vi "point-picker.vi"() -> ()   [LabVIEW 2013]
uses:
  <vilib>/Utility/file.llb/Read From Spreadsheet File (DBL).vi
panel:
  out "X Scale.Range:Minor Increment":dbl=0.00010000000000000009
  out "Slice":dbl[](graph)=[0.03882083763653586, 0.036301990430997515, 0.06641265033129048, 0.022599259175726628, 0.03963233726656525, 0.057976093950650155, 0.02605338207009137, 0.04157947175893252, 0.008818364898812232, 0.03339557369538179, 0.009831003676912626, 0.0298513507596618, 0.000720265042160115, 0.04957020405641017, 0.028435297883295477, 0.02968065104257011, 0.054593725454568406, 0.02941844990660442, 0.0016610067970859927, 0.037814320441856994, 0.03162073969486945, 0.04354178631802414, 0.01837108453843325, 0.020494923878462044, 0.02146464095599344, 0.050724892633311223, 0.055113319254019744, 0.010244418203584982, 0.02498233101668227, 0.02800231949963939, 0.02428971264494624, 0.03964718893141746, 0.03696606646661389, 0.04173575239047644, 0.08038701264805279, 0.05693297539500711, 0.031549742745971894, 0.010177653448556319, 0.047274462597502925, 0.018015425707227962, 0.032278808272603966, 0.04953827011027471, 0.06425909702809958, 0.018330341600943854, 0.03463798404659602, 0.03930752357841345, 0.06796427722786236, 0.02058242219084138, 0.04370799015223786, 0.023590787930164128, 0.008461873502233855, 0.029360130887503208, 0.029158674398922235, 0.03945732345450104, 0.012916360547716334, 0.02759490800230026, 0.03753745241666211, 0.028389751605858184, 0.0150134372573898, 0.009742076686166182, 0.019301765168510596, 0.017192190302683024, 0.037235678285443434, 0.011830534813551296, 0.002788759120713905, 0.047997520126393176, 0.030486497700197693, 0.0546373685612716, 0.033694598255554375, 0.07210813163063974, 0.0698476088075215, 0.05675370368842305, 0.018003794508399205, 0.05840152492070653, 0.07904339321982226, 0.01935226022484138, 0.02798406675494754, 0.040280610248166655, 0.03827329030370933, 0.05730522884686868, 0.028632706255257163, 0.03808138034326173, 0.023911063204232516, 0.02860009511132246, 0.03013417630372773, 0.05786997254233813, 0.034379154781915416, 0.057090706930711166, 0.0065538518251016305, 0.034942872579625674, 0.04085803640097609, 0.05948489786153084, 0.016636040413519484, 0.044311424683074925, 0.011781703345063444, 0.03242739475202488, 0.03446934597584147, 0.019995898772222725, 0.03788022352986928, 0.07073965157227771, 0.0484240053769007, 0.02956512492392868, 0.03343667145168942, 0.048772763779949456, 0.023260771689348297, 0.024232846201902924, 0.01926514322840278, 0.04281073931274156, 0.012469809763181561, 0.0641590005902021, 0.01036489387193246, 0.023713733127830185, 0.003418705886296209, 0.005247242164587641, 0.05102637721139735, 0.017050054644982493, 0.038652476635340084, 0.0755487811686583, 0.03302481941271952, 0.027735460779743856, 0.00891767772967212, 0.0398685162454713, 0.05828907527641214, 0.04695682915759623, 0.04187443482881026, 0.029803188979993425, 0.031115433917284076, 0.03570030269691735, 0.013937499423103702, 0.026584094060496527, 0.023214915238454457, 0.027620529801687166, 0.03216913388862226, 0.026476641423870587, 0.03544898608213742, 0.013068897496967921, 0.030785916593722085, 0.08446811893320971, 0.3808105906232525, 0.6572630448339808, 0.3660975082961466, 0.021944554366762136, 0.01953504034414964, 0.04781580361655588, 0.04160295903297597, 0.05916878461180063, 0.027743208538463692, 0.0349214596482308, 0.009739236772262355, 0.035293979346204506, 0.03332222838294596, 0.03917347835627661, 0.011226281764677612, 0.046852750781702084, 0.02682215429743462, 0.02459883098718702, 0.03745736029631423, 0.037909602739041946, 0.0046436282813863425, 0.0071526550619555596, 0.06169741653962818, 0.037594249281427614, 0.02157475809520118, 0.05768831217094244, 0.07269251067649998, 0.04469432097642645, 0.0405574904531571, 0.04998481804236441, 0.02201281282476729, 0.029448012231665262, 0.0344571687459247, 0.05233290045359092, 0.017807686687307613, 0.0704820989294821, 0.06281436676107005, 0.05569904973473387, 0.06667145542210462, 0.050083393220346016, 0.06288651353602691, 0.10651812416066751, 0.10390581812121322, 0.18618470866578526, 0.20944068902059454, 0.3330231646021931, 0.4068341589920195, 0.557518984228075, 0.6722771293285174, 0.7705694411559676, 0.7136035014113573, 0.456773566237813, 0.32679353287086677, 0.17469742643513897, 0.11241662421216703, 0.05711150001827489, 0.05684758198913661, 0.058197453071294765, 0.08088584025205328, 0.028661415628547682, 0.06533929361633121, 0.057882789502990306, 0.019948090213825955, 0.028398676423295445, 0.022590854443279254, 0.038127041664969795, 0.022098100031424036, 0.019914607931659573, 0.03462224359590756, 0.029590831640898714, 0.01876528543540782, 0.05403197264262346, 0.01820980358237397, 0.03262754592585054, 0.039328214102196064, 0.02001116355072607, 0.046825409437886656, 0.024195009961849742, 0.01174278792531118, 0.013228660257657709, 0.04323872349673986, 0.016618521721934353, 0.029778228383874235, 0.03790569531420866, 0.039550584490196654, 0.019345730579277045, 0.04533889119133574, 0.04122424012659842, 0.010797084585577587, 0.010475681550390591, 0.005625118452838267, 0.018411178614552187, 0.03902153594714584, 0.0476843406427223, 0.021005695266023375, 0.02524771788840599, 0.01605204219736099, 0.03854728236804991, 0.02601656693340934, 0.05085858012862036, 0.04249344660781145, 0.05237586835447254, 0.03546830423867645, 0.03549050530059798, 0.013858786818514112, 0.04242378496354003, 0.004401079825498598, 0.04720662808781359, 0.01232274436915387, 0.016105856205135844, 0.03881904383723042, 0.03422196329298994, 0.0311331546633088, 0.03245000370099103, 0.04009676368174022, 0.054023538400867405, 0.03482918134608338, 0.045505865937143106, 0.05440485965682107, 0.021641566970397437, 0.07229965735776268, 0.02411390238224905, 0.037334738585570106, 0.045371115366053226, 0.029103996301753268, 0.041528882691374815, 0.018358973440157595, 0.016688411720087813, 0.006528885247806317, 0.05168244948458969, 0.03710184786373036, 0.024124982205265138, 0.040078292861693086, 0.023156562614362206, 0.02745180608419872, 0.021613183443570192, 0.03495913949543546, 0.007448621323276699, 0.04507216597376568, 0.026398651880534862, 0.008678370927622723, 0.0050946707642497355, 0.04908065606338803, 0.047045493087371194, 0.014933947276883627, 0.047943308180870316, 0.04228377247645035, 0.029255550479048282, 0.04206501038954848, 0.04466146482600919, 0.055006090493927594, 0.03175612304150846, 0.06174627790201885, 0.023461899834064163, 0.013568954299388366, 0.024545963323765893, 0.0208250573877551, 0.05134103259107603, 0.024065567710157658, 0.03165014064060575, 0.01825012772750901, 0.03249082063226778, 0.026998952799489637, 0.02181659322762004, 0.04137283667622604, 0.028319134745111847, 0.040495847881314544, 0.0425882578154225, 0.05367681909024711, 0.06449946446549276, 0.028254662736405624, 0.023366607192255407, 0.03812310895281717, 0.05943609515620472, 0.04855506102140248, 0.01972053585653053, 0.08437300454694428, 0.021958724677403067, 0.03310082653278058, 0.0041907814881053974, 0.03087300810539439, 0.03175668555037808, 0.07593033993572323, 0.02067213276715719, 0.014832946676285708, 0.04836684450377593, 0.02035005458379112, 0.03923147171547854, 0.04083944885831917, 0.01650058281029404, 0.03998571696531034, 0.026012636117049293, 0.011082093219741636, 0.04011572369488455, 0.0484420604511582, 0.04033404621138865, 0.06151817442991706, 0.020275548131516306, 0.03041005829657886, 0.02679158631048964, 0.020932226243095552, 0.07054258780039666, 0.024135088294546532, 0.016138203870400325, 0.023556247185348368, 0.013230797094894728, 0.012996564511889035, 0.03935096998244559, 0.02141118457848609, 0.037980080089989425, 0.017687346529578887, 0.02453612091543529, 0.0511699853014372, 0.04581895281912373, 0.05906906624438031, 0.032438148270553774, 0.018783429090892003, 0.029307845448098783, 0.032419276281024305, 0.0716498115963489, 0.07245208637243722, 0.04081598634816035, 0.06809892094827617, 0.018452956950161758, 0.02792326968864213, 0.04393413610648986, 0.05269399277500646, 0.03229624331169929, 0.03459551738390979, 0.05687054706417872, 0.04157074130736018, 0.05105338889165303, 0.0592684995837126, 0.01952377961244403, 0.04113450814463985, 0.04052194087956064, 0.04111246149225709, 0.020407157507984244, 0.06719307569344483, 0.05645228148763298, 0.04191832866122989, 0.022633650815248745, 0.06474175777733716, 0.007421439755066878, 0.035907099643956795, 0.05000776269158416, 0.0324420291173828, 0.03733168950938588, 0.0572035357046293, 0.01652732875809153, 0.04390532569322737, 0.07135619168333725, 0.027028090462443338, 0.031108350063770395, 0.06642566760942425, 0.011214809917434178, 0.057874702289397395, 0.04267403621074702, 0.007668307109211589, 0.059114791994878, 0.01912389632385104, 0.014625408574295264, 0.06856776851688241, 0.05958030479400584, 0.0560114723877861, 0.044960222053147564, 0.0503632587886607, 0.033851940532008344, 0.04904636141470431, 0.04912762163574193, 0.023723692707653708, 0.03867405670468051, 0.022703402976533633, 0.09313612277194461, 0.10751243146099411, 0.029319266466846503, 0.04846783515663733, 0.05538798855719933, 0.09243049914095047, 0.025090894008307888, 0.0341597087940961, 0.08102638609307984, 0.026597051167136527, 0.034553152154660115, 0.07806219820738826, 0.020339039917854747, 0.027792448560806742, 0.035276027967281395, 0.015842617199590008, 0.021079657904548105, 0.06674918670325417, 0.0384203833635449, 0.044497107493775674, 0.04846289790808542, 0.04335897137600318, 0.057869233631084795, 0.0213879914703754, 0.04793177850709304, 0.046860022502610746, 0.029004201961304245, 0.048816060786727886, 0.05118992770319197, 0.038939794329080124, 0.08243147020908992, 0.0179638231025117, 0.04136424345135459, 0.049899963216828616, 0.08163456016429607, 0.0795608619209012, 0.01797972488165152, 0.07141519168495342, 0.05081509773883891, 0.0481149686266734, 0.06279110670293864, 0.044376948207529576, 0.0714076617516406, 0.07836812113934964, 0.059317556888100864, 0.016492944764773473, 0.011355573443542731, 0.06768871545737691, 0.04009394308159768, 0.07418289329424736, 0.0604651039233088, 0.05480586504842359, 0.0796076289393417, 0.022972728268496792, 0.06297259609675009, 0.07702589272289448, 0.03664220371316584, 0.04387637160195887, 0.06633068528810106, 0.07473871733104656, 0.015268628544294999, 0.061861002412350236, 0.06830575773316326, 0.01642782862084517, 0.06275029133553639, 0.0695148118689358, 0.041423519966301475, 0.040194172424721446, 0.07606286406281303, 0.055888985232942105, 0.052318268059792485, 0.06896599647465837, 0.08490319833193526, 0.03711139233108567, 0.015997146890139858, 0.04661373867578224, 0.012622281818933224, 0.024831215965328144, 0.08643492530910662, 0.06577904647233777, 0.029884568725016422, 0.06773798968762446, 0.04199281688167392, 0.07218541874847897, 0.02253846517094748, 0.0682131686355302, 0.029028784585931215, 0.06052229397409447, 0.05226875063818199, 0.023568866395418546]
  in  "Load From File!":bool
  in  "File":path=path "C:/ExperimentBlue/2021-03-16_transmon-with-filter/2021-03-17_transmon-with-filter_010_q4-2tone-detailed.txt"
  in  "Up":bool
  in  "Down":bool
  in  "Shift y":dbl=2000000.0 step=200000.0 format="%#_6p"
  in  "Shift x":dbl=0.00010000000000000009 step=1.000000000000001e-05
  in  "Move":bool
  in  "Select":bool
  in  "Boolean":bool
  out "Y-Position":dbl=9242989473.68421
  out "X-Position":dbl=0.04760257731958763
  in  "Subtract_Amp":dbl[][](graph)=array51x501[25551 elements]
  out "X Array":dbl[](array[numeric])
  out "Y Array":dbl[](array[numeric])
  out "Picked Points":cluster{dbl[], dbl[]}(graph)
  # "Drop it here -> create refference and connect on block diagram"
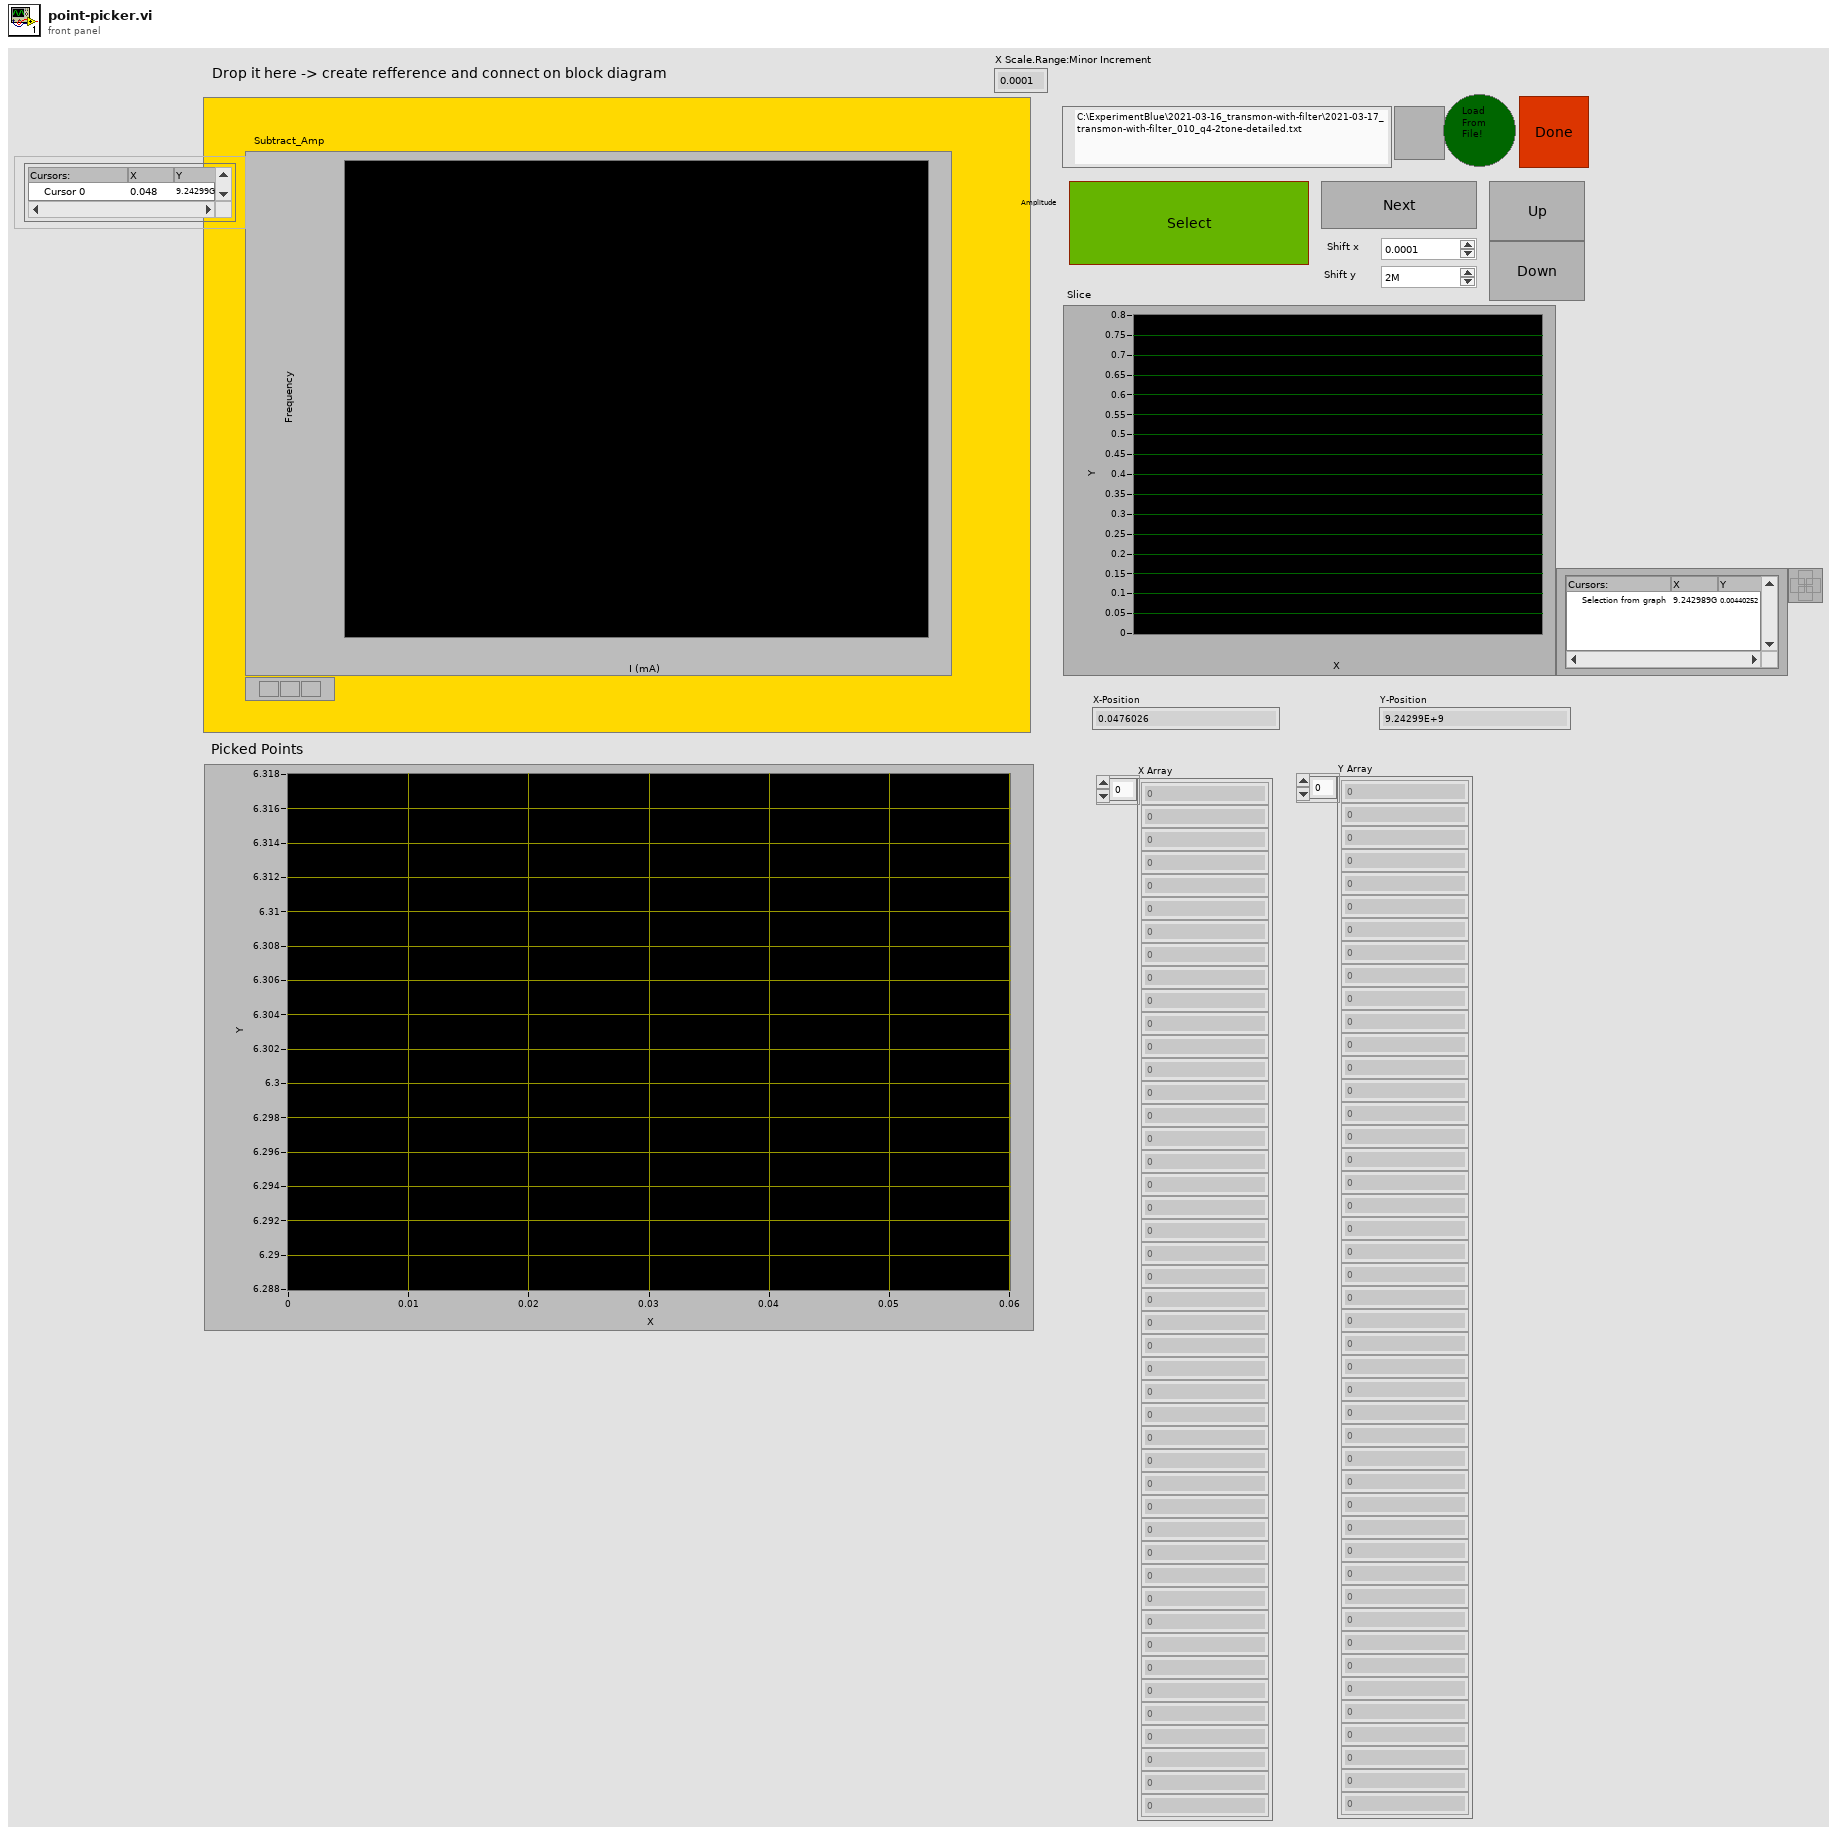
[diagram p1: front panel]
types:
  T1 = enum16{"open", "replace", "create", "open or create", "replace or create", "replace or create with confirmation"}
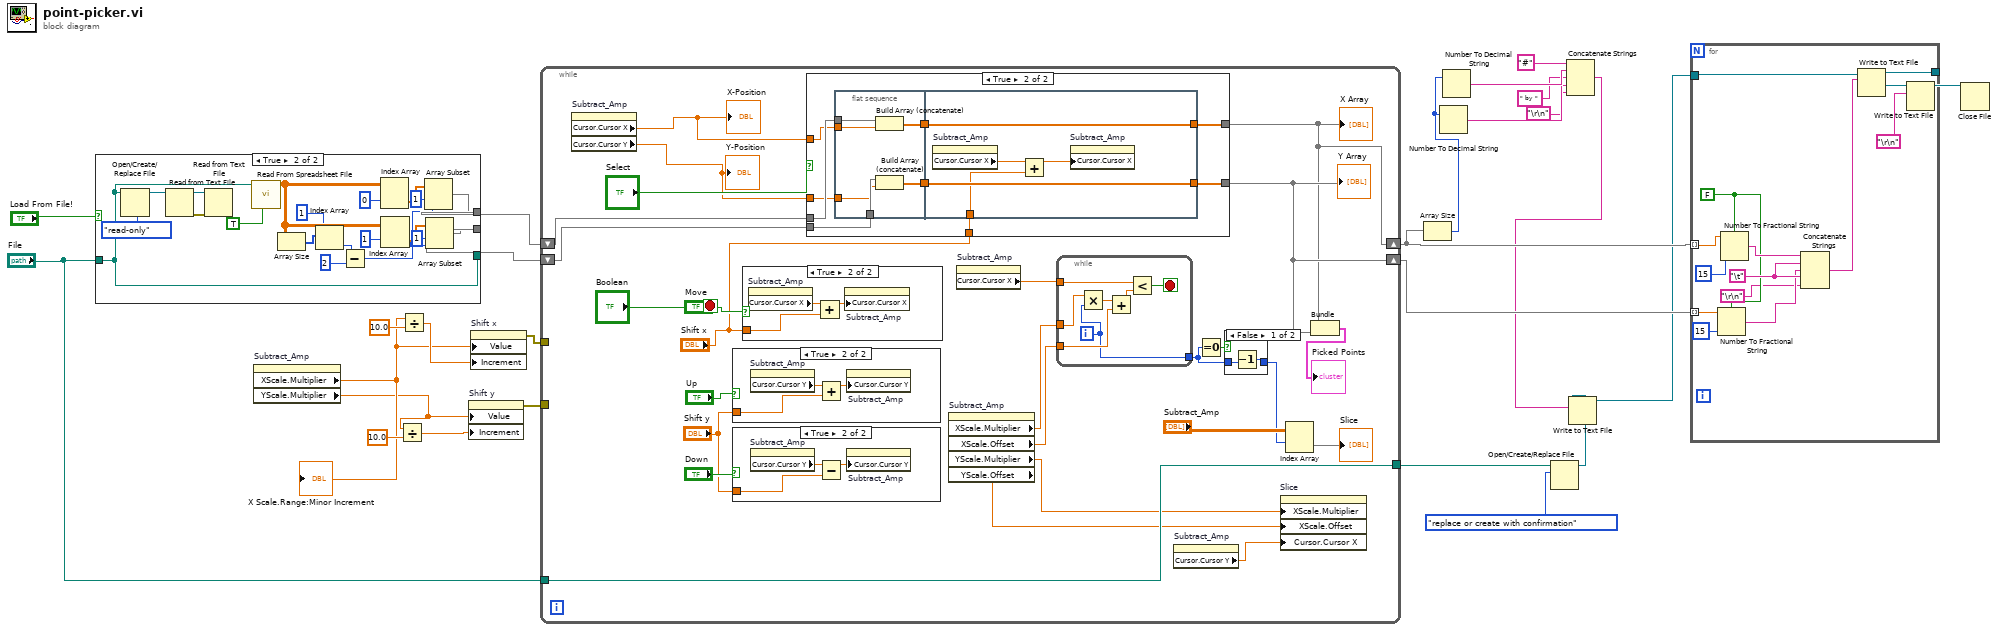
[diagram p0: block diagram]
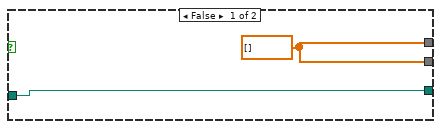
[diagram p2: hidden frame]
diagram:
  n1 = case shown="True" "Load From File!" {
    tunnel: [w30 w46] -> _
    tunnel: "File" -> [w30 w46]
    tunnel: [w29 w38] -> w15
    tunnel: [w29 w37] -> w14
    frame False {
      w29 = dbl[] []
    }
    frame True {
      n2 = Open/Create/Replace File(file path (use dialog)=w46, access (0:read/write)=enum16{"read/write", "read-only", "write-only"}."read-only") -> (refnum out=w49:refnum<file>)  [unwired: 4 in, 2 out]
      n3 = Read from Text File(file (use dialog)=w49) -> (refnum out=w47:refnum<file>, error out=w48:errorcluster)  [unwired: 3 in, 2 out]
      n4 = Read from Text File(file (use dialog)=w47, error in=w48) -> ()  [unwired: 2 in, 4 out]
      n5 = call-poly <vilib>:"Read From Spreadsheet File.vi"("transpose (no:F)"=TRUE, "file path (dialog if empty)"=w46) -> ("all rows"=w36:dbl[][])  [unwired: 5 in, 4 out]
      n6 = Array Size(array=w36) -> (size(s)=w35:i32[])
      n7 = Index Array(array=w35, index=1) -> (element=w33:i32)
      n8 = Subtract(x=w33, y=2) -> (x-y=w31:i32)
      n9 = Index Array(array=w36, index (row)=0) -> (element=w43:dbl[])  [unwired: 1 in]
      n10 = Index Array(array=w36, index (row)=1) -> (element=w40:dbl[])  [unwired: 1 in]
      n11 = Array Subset(array=w43, index=1, length=w31) -> (w38:dbl[])
      n12 = Array Subset(array=w40, index=1, length=w31) -> (w37:dbl[])
    }
  }
  n13 = property on="Subtract_Amp" class="IntGraph (strict)"() -> ("XScale.Multiplier"=w23:dbl, "YScale.Multiplier"=w22:dbl)  [unwired: 2 in, 2 out]
  "X Scale.Range:Minor Increment" <- w23
  n14 = Divide(x=w22, y=10.0) -> (x/y=w21:dbl)
  n15 = Divide(x=w23, y=10.0) -> (x/y=w24:dbl)
  n16 = property on="Shift y" class="DigNum (strict)"("Value"=w22, "Increment"=w21) -> (error out=w19:errorcluster)  [unwired: 2 in, 1 out]
  n17 = property on="Shift x" class="DigNum (strict)"("Value"=w23, "Increment"=w24) -> (error out=w20:errorcluster)  [unwired: 2 in, 1 out]
  n18 = while {
    shift-right: [w65] -> w27
    shift-left: w14 -> [w74]
    shift-right: [w62] -> w28
    shift-left: w15 -> [w73]
    tunnel: w20 -> [_]
    tunnel: w19 -> [_]
    tunnel: [w63] -> w18
    tunnel: "File" -> [w63]
    stop <- "Boolean" stop-if-true
    n19 = property on="Subtract_Amp" class="IntGraph (strict)"() -> ("Cursor.Cursor X"=w72:dbl, "Cursor.Cursor Y"=w71:dbl)  [unwired: 2 in, 2 out]
    "X-Position" <- w72
    "Y-Position" <- w71
    n20 = case shown="True" "Up" {
      tunnel: "Shift y" -> [_ w92]
      frame False {
      }
      frame True {
        n21 = property on="Subtract_Amp" class="IntGraph (strict)"() -> ("Cursor.Cursor Y"=w91:dbl)  [unwired: 2 in, 2 out]
        n22 = Add(x=w91, y=w92) -> (x+y=w90:dbl)
        n23 = property on="Subtract_Amp" class="IntGraph (strict)"("Cursor.Cursor Y"=w90) -> ()  [unwired: 2 in, 2 out]
      }
    }
    n24 = case shown="True" "Down" {
      tunnel: "Shift y" -> [_ w89]
      frame False {
      }
      frame True {
        n25 = property on="Subtract_Amp" class="IntGraph (strict)"() -> ("Cursor.Cursor Y"=w88:dbl)  [unwired: 2 in, 2 out]
        n26 = Subtract(x=w88, y=w89) -> (x-y=w87:dbl)
        n27 = property on="Subtract_Amp" class="IntGraph (strict)"("Cursor.Cursor Y"=w87) -> ()  [unwired: 2 in, 2 out]
      }
    }
    n28 = case shown="True" "Move" {
      tunnel: "Shift x" -> [_ w95]
      frame False {
      }
      frame True {
        n29 = property on="Subtract_Amp" class="IntGraph (strict)"() -> ("Cursor.Cursor X"=w94:dbl)  [unwired: 2 in, 2 out]
        n30 = Add(x=w94, y=w95) -> (x+y=w93:dbl)
        n31 = property on="Subtract_Amp" class="IntGraph (strict)"("Cursor.Cursor X"=w93) -> ()  [unwired: 2 in, 2 out]
      }
    }
    n32 = case shown="True" "Select" {
      tunnel: w74 -> [w96 w103]
      tunnel: w73 -> [w97 w106]
      tunnel: w72 -> [_ w105]
      tunnel: [w97 w104] -> w62
      tunnel: w71 -> [_ w102]
      tunnel: [w96 w101] -> w65
      tunnel: "Shift x" -> [_ w98]
      frame False {
      }
      frame True {
        n33 = flat-sequence {
          tunnel: w106 -> [w112]
          tunnel: w105 -> [w111]
          tunnel: w103 -> [w109]
          tunnel: w102 -> [w108]
          tunnel: [w110] -> w100
          tunnel: [w107] -> w99
          tunnel: [w116] -> w101
          tunnel: [w117] -> w104
          tunnel: w100 -> [w117]
          tunnel: w99 -> [w116]
          tunnel: w98 -> [w113]
          frame #0 {
            n34 = Build Array (concatenate)(w112, w111) -> (w110:dbl[])
            n35 = Build Array (concatenate)(w109, w108) -> (w107:dbl[])
          }
          frame #1 {
            n36 = property on="Subtract_Amp" class="IntGraph (strict)"() -> ("Cursor.Cursor X"=w114:dbl)  [unwired: 2 in, 2 out]
            n37 = Add(x=w114, y=w113) -> (x+y=w115:dbl)
            n38 = property on="Subtract_Amp" class="IntGraph (strict)"("Cursor.Cursor X"=w115) -> ()  [unwired: 2 in, 2 out]
          }
        }
      }
    }
    "Y Array" <- w65
    "X Array" <- w62
    n39 = property on="Subtract_Amp" class="IntGraph (strict)"() -> ("XScale.Multiplier"=w59:dbl, "XScale.Offset"=w58:dbl, "YScale.Multiplier"=w57:dbl, "YScale.Offset"=w56:dbl)  [unwired: 2 in, 2 out]
    n40 = property on="Subtract_Amp" class="IntGraph (strict)"() -> ("Cursor.Cursor X"=w54:dbl)  [unwired: 2 in, 2 out]
    n41 = while {
      tunnel: w54 -> [w85]
      tunnel: w59 -> [w86]
      tunnel: w58 -> [w83]
      tunnel: [w81] -> w51
      i -> [w81]
      stop <- w80 stop-if-true
      n42 = Multiply(x=w86, y=w81) -> (x*y=w82:dbl)
      n43 = Add(x=w82, y=w83) -> (x+y=w84:dbl)
      n44 = Less?(x=w85, y=w84) -> (x < y?=w80:bool)
    }
    n45 = property on="Subtract_Amp" class="IntGraph (strict)"() -> ("Cursor.Cursor Y"=w55:dbl)  [unwired: 2 in, 2 out]
    n46 = Equal To 0?(x=w51) -> (x = 0?=w53:bool)
    n47 = case shown="False" w53 {
      tunnel: [w78 w79] -> w52
      tunnel: w51 -> [w77 w79]
      frame False {
        n48 = Decrement(x=w77) -> (x-1=w78:i32)
      }
      frame True {
      }
    }
    n49 = property on="Slice" class="WFGraph (strict)"("XScale.Multiplier"=w57, "XScale.Offset"=w56, "Cursor.Cursor X"=w55) -> ()  [unwired: 2 in, 2 out]
    n50 = Index Array(array="Subtract_Amp", index (row)=w52) -> (element=→"Slice":dbl[])  [unwired: 1 in]
    n51 = Bundle(w62, w65) -> (→"Picked Points":cluster{dbl[], dbl[]})  [unwired: 1 in]
  }
  n52 = Array Size(array=w28) -> (size(s)=w5:i32)
  n53 = Number To Decimal String(number=w5) -> (decimal integer string=w8:string)  [unwired: 1 in]
  n54 = Number To Decimal String(number=w5) -> (decimal integer string=w10:string)  [unwired: 1 in]
  n55 = Open/Create/Replace File(file path (use dialog)=w18, operation (0:open)=T1."replace or create with confirmation") -> (refnum out=w1:refnum<file>)  [unwired: 4 in, 2 out]
  n56 = Concatenate Strings("#" ("string"), w10, " by " ("string"), w8, "\r\n") -> (w4:string)
  n57 = Write to Text File(file (use dialog)=w1, text=w4) -> (refnum out=w3:refnum<file>)  [unwired: 2 in, 2 out]
  n58 = for {
    tunnel: w3 -> [w129]
    tunnel: [w125] -> w11
    tunnel: w28 -> [w121] mode=indexing
    tunnel: w27 -> [w120] mode=indexing
    w122 = FALSE ("use system decimal point (T)")
    w127 = "\t"
    n59 = Number To Fractional String(use system decimal point (T)=w122, number=w120, precision (6)=i16 15) -> (F-format string=w119:string)  [unwired: 1 in]
    n60 = Number To Fractional String(use system decimal point (T)=w122, number=w121, precision (6)=i16 15) -> (F-format string=w128:string)  [unwired: 1 in]
    n61 = Concatenate Strings(w128, w127, w119, w127, "\r\n") -> (w126:string)
    n62 = Write to Text File(file (use dialog)=w129, text=w126) -> (refnum out=w125:refnum<file>)  [unwired: 2 in, 2 out]
  }
  n63 = Write to Text File(file (use dialog)=w11, text="\r\n") -> (refnum out=w12:refnum<file>)  [unwired: 2 in, 2 out]
  n64 = Close File(refnum=w12) -> ()  [unwired: 1 in, 2 out]
